vi "lv-ros-bridge_WRITE.vi"(10 "rosbridge port":u16=9090, 11 "rosbridge server IP":string="192.168.164.128") -> (0 "error out":errorcluster)   [LabVIEW 2015]
uses:
  Control  rossss.ctl
  <vilib>/Utility/inputDevices.llb/joystickAcquire.vi
  <vilib>/Utility/inputDevices.llb/closeJoystick.vi
  <vilib>/Intelligent Energy/WebSockets API/WebSockets/WebSockets.lvlib
panel:
  in  "ms to wait":u32=10
  in  "msg.layout.dim":T1(array[cluster])
  out "output cluster":T2={"op"="publish", "topic"="", "msg"={"layout"={"dim"=[], "data_offset"=0.0}, "data"=[]}}
  out "Opcode 2":u8
  out "Data 2":string
  out "concatenated string":string
  in  "type":string="std_msgs/Int32MultiArray"
  out "direction info":T3
  out "button info":T4
  out "axis info":T5
  in  "device index":i32
  in  "Topic to write":string="rio"
  in  "format wiadomości":T2={"op"="publish", "topic"="", "msg"={"layout"={"dim"=[], "data_offset"=0.0}, "data"=[]}}
  out "raw JSON frame":string
  in  "stop":bool
  # "ZAWSZE UŻYWAJ STOPU!!!"
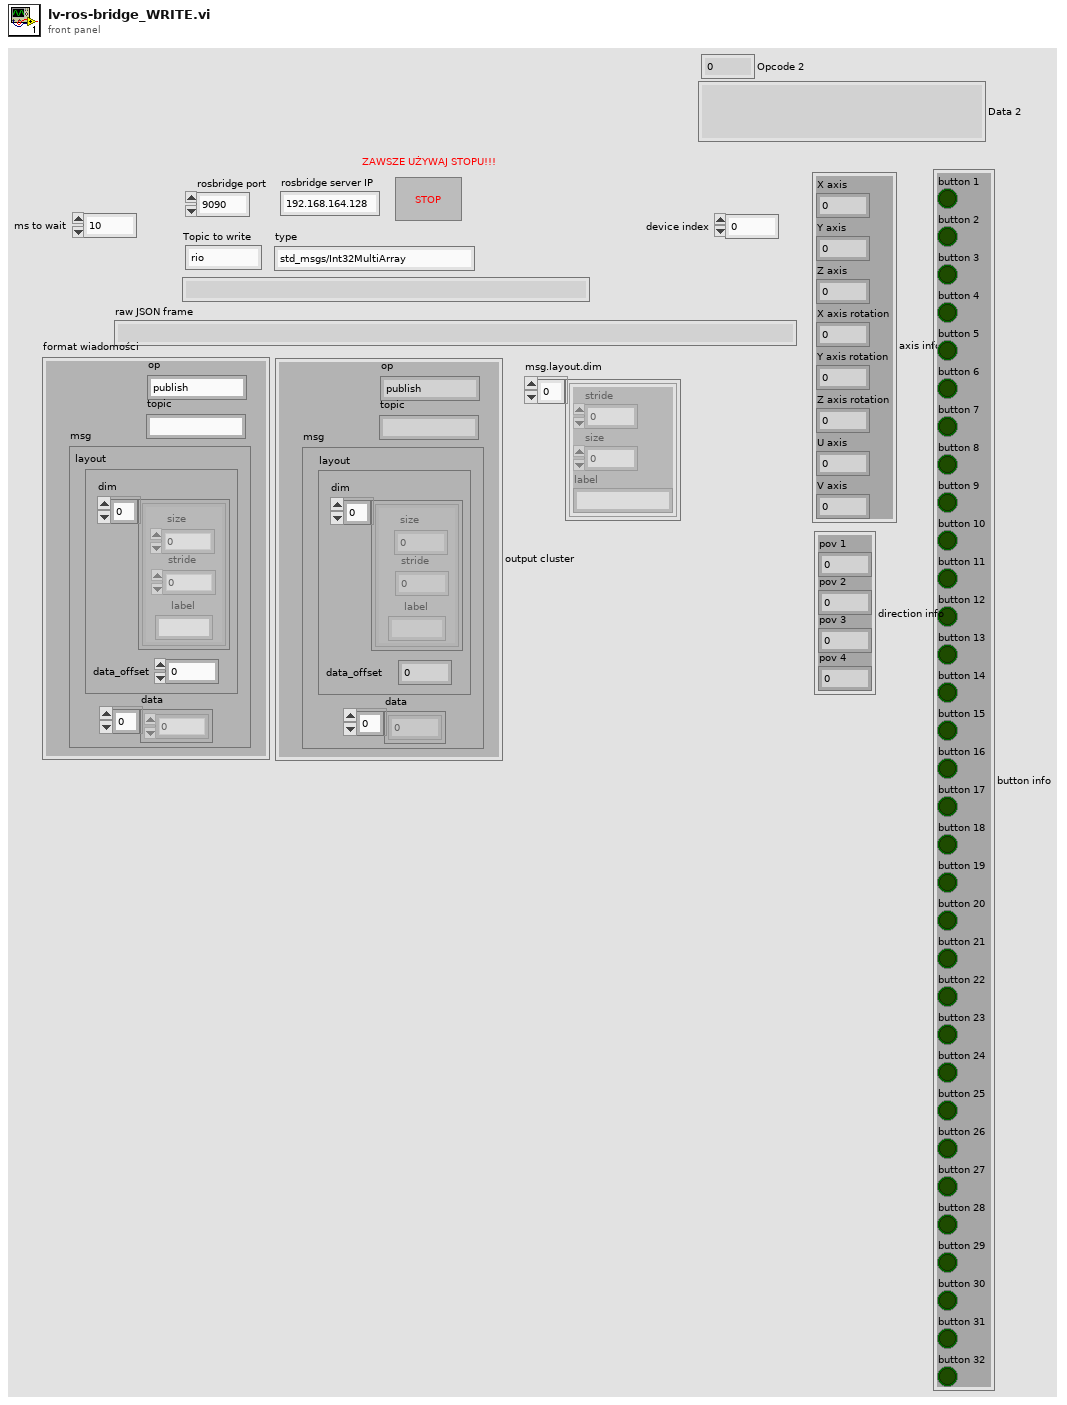
[diagram p1: front panel]
types:
  T1 = cluster{"stride":i16, "size":i16, "label":string}[]
  T2 = typedef "Control  rossss.ctl" = cluster{"op":string, "topic":string, "msg":cluster{"layout":cluster{"dim":cluster{"stride":i16, "size":i16, "label":string}[], "data_offset":dbl}, "data":i32[]}}
  T3 = cluster{"pov 1":i32, "pov 2":i32, "pov 3":i32, "pov 4":i32}
  T4 = cluster{"button 1":bool, "button 2":bool, "button 3":bool, "button 4":bool, "button 5":bool, "button 6":bool, "button 7":bool, "button 8":bool, "button 9":bool, "button 10":bool, "button 11":bool, "button 12":bool, "button 13":bool, "button 14":bool, "button 15":bool, "button 16":bool, "button 17":bool, "button 18":bool, "button 19":bool, "button 20":bool, "button 21":bool, "button 22":bool, "button 23":bool, "button 24":bool, "button 25":bool, "button 26":bool, "button 27":bool, "button 28":bool, "button 29":bool, "button 30":bool, "button 31":bool, "button 32":bool}
  T5 = cluster{"X axis":i32, "Y axis":i32, "Z axis":i32, "X axis rotation":i32, "Y axis rotation":i32, "Z axis rotation":i32, "U axis":i32, "V axis":i32}
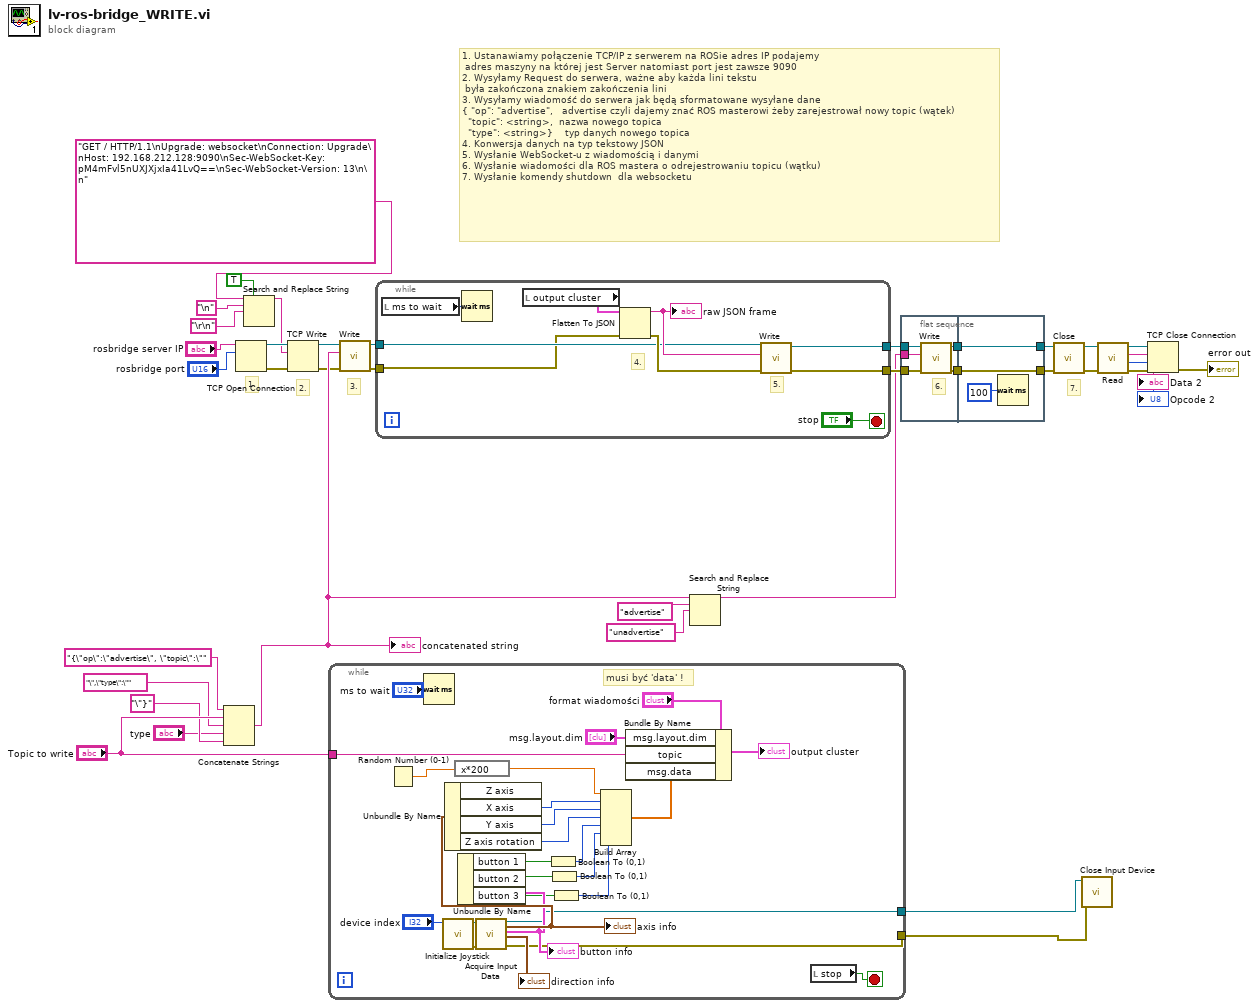
[diagram p0: block diagram]
diagram:
  # "1. Ustanawiamy połączenie TCP/IP z serwerem na ROSie adres IP podajemy\n adres maszyny na której jest Server natomiast port jest zawsze 9090\n2. Wysyłamy Request do serwera, ważne aby każda lini tekstu\n była zakończona znakiem zakończenia lini\n3. Wysyłamy wiadomość do serwera jak będą sformatowane wysyłane dane \n{ \"op\": \"advertise\",   advertise czyli dajemy znać ROS masterowi żeby zarejestrował nowy topic (wątek)\n  \"topic\": <string>,  nazwa nowego topica \n  \"type\": <string>}    typ danych nowego topica\n4. Konwersja danych na typ tekstowy JSON\n5. Wysłanie WebSocket-u z wiadomością i danymi\n6. Wysłanie wiadomości dla ROS mastera o odrejestrowaniu topicu (wątku)\n7. Wysłanie komendy shutdown  dla websocketu"
  # "7."
  # "3."
  # "2."
  # "1."
  n1 = Concatenate Strings("{\"op\":\"advertise\", \"topic\":\"", "Topic to write", "\",\"type\":\"", "type", "\"}") -> (w32:string)
  "concatenated string" <- w32
  n2 = TCP Open Connection(address="rosbridge server IP", remote port or service name="rosbridge port") -> (connection ID=w14:refnum<k5>, error out=w13:errorcluster)  [unwired: 3 in]
  n3 = Search and Replace String(replace all?=TRUE ("replace all? (F)"), input string="GET / HTTP/1.1\nUpgrade: websocket\nConnection: Upgrade\nHost: 192.168.212.128:9090\nSec-WebSocket-Key: pM4mFvl5nUXJXjxIa41LvQ==\nSec-WebSocket-Version: 13\n\n", search string="\n", replace string="\r\n") -> (result string=w12:string)  [unwired: 4 in, 3 out]
  n4 = TCP Write(connection ID=w14, data in=w12, error in (no error)=w13) -> (connection ID out=w2:refnum<k5>, error out=w1:errorcluster)  [unwired: 1 in, 1 out]
  n5 = while {
    tunnel: "Topic to write" -> [w61]
    tunnel: [w44] -> w31
    tunnel: [w43] -> w30
    stop <- w62 stop-if-true
    # "musi być 'data' !"
    n6 = Random Number (0-1)() -> (number: 0 to 1=w39:dbl)
    n7 = Wait (ms)(milliseconds to wait="ms to wait") -> ()  [unwired: 1 out]
    n8 = call <vilib>:"Initialize Joystick.vi"("device index"="device index") -> ("error out"=w56:errorcluster, "device ID"=w57:refnum<k1>)  [unwired: 9 in]
    n9 = expression code="x*200"(w39) -> (w38:dbl)
    n10 = call-poly <vilib>:"Acquire Input Data.vi"("device ID"=w57, "error in (no error)"=w56) -> ("device ID"=w44:refnum<k1>, "axis info"=w55:T5, "button info"=w51:T4, "direction info"=→"direction info":T3, "error out"=w43:errorcluster)  [unwired: 13 in]
    "axis info" <- w55
    "button info" <- w51
    n11 = Unbundle By Name(w55) -> ("X axis"=w54:i32, "Y axis"=w53:i32, "Z axis rotation"=w52:i32)  [unwired: 1 out]
    n12 = Unbundle By Name(w51) -> ("button 1"=w48:bool, "button 2"=w49:bool, "button 3"=w50:bool)
    n13 = Boolean To (0,1)(Boolean=w48) -> (0, 1=w47:i16)
    n14 = Boolean To (0,1)(Boolean=w49) -> (0, 1=w46:i16)
    n15 = Boolean To (0,1)(Boolean=w50) -> (0, 1=w45:i16)
    n16 = Build Array(w38, w54, w53, w52, w47, w46, w45) -> (w41:dbl[])
    n17 = Bundle By Name(cluster="format wiadomości", "msg.layout.dim"="msg.layout.dim", "topic"=w61, "msg.data"=w41) -> (→"output cluster":T2)
    n18 = local read "stop"() -> (w62:bool)
  }
  n19 = call <vilib>:"Write.vi"("error in (no error)"=w1, "Data"=w32, "WebSocket Connection in"=w2) -> ("error out"=w26:errorcluster, "WebSocket Connection out"=w25:refnum<k5>)  [unwired: 7 in]
  n20 = while {
    tunnel: [w72] -> w23
    tunnel: [w71] -> w21
    tunnel: w25 -> [w66]
    tunnel: w26 -> [w65]
    stop <- "stop" stop-if-true
    # "5."
    # "4."
    n21 = local read "ms to wait"() -> (w64:u32)
    n22 = Wait (ms)(milliseconds to wait=w64) -> ()  [unwired: 1 out]
    n23 = local read "output cluster"() -> (w68:T2)
    n24 = Flatten To JSON(anything=w68, error in (no error)=w65) -> (JSON string=w69:string, 11:w67:errorcluster)  [unwired: 1 in]
    "raw JSON frame" <- w69
    n25 = call <vilib>:"Write.vi"("error in (no error)"=w67, "Data"=w69, "WebSocket Connection in"=w66) -> ("error out"=w71:errorcluster, "WebSocket Connection out"=w72:refnum<k5>)  [unwired: 7 in]
  }
  n26 = Search and Replace String(input string=w32, search string="advertise", replace string="unadvertise" ("search string")) -> (result string=w11:string)  [unwired: 5 in, 3 out]
  n27 = flat-sequence {
    tunnel: w23 -> [w77]
    tunnel: w21 -> [w76]
    tunnel: w11 -> [w75]
    tunnel: [w74] -> w29
    tunnel: [w73] -> w28
    tunnel: [w79] -> w22
    tunnel: [w80] -> w24
    tunnel: w29 -> [w80]
    tunnel: w28 -> [w79]
    frame #0 {
      # "6."
      n28 = call <vilib>:"Write.vi"("error in (no error)"=w76, "Data"=w75, "WebSocket Connection in"=w77) -> ("error out"=w73:errorcluster, "WebSocket Connection out"=w74:refnum<k5>)  [unwired: 7 in]
    }
    frame #1 {
      n29 = Wait (ms)(milliseconds to wait=u32 100) -> ()  [unwired: 1 out]
    }
  }
  n30 = call <vilib>:"Close.vi"("error in (no error)"=w22, "WebSocket Connection in"=w24) -> ("error out"=w7:errorcluster, "WebSocket Connection in"=w8:refnum<k5>)  [unwired: 8 in]
  n31 = call-poly <vilib>:"Close Input Device.vi"("error in (no error)"=w30, "device ID"=w31) -> ()  [unwired: 8 in, 1 out]
  n32 = call <vilib>:"Read.vi"("error in (no error)"=w7, "WebSocket Connection in"=w8) -> ("error out"=w6:errorcluster, "Opcode"=→"Opcode 2":u8, "Data"=→"Data 2":string, "WebSocket Connection out"=w5:refnum<k5>)  [unwired: 6 in]
  n33 = TCP Close Connection(connection ID=w5, error in (no error)=w6) -> (error out=→"error out":errorcluster)  [unwired: 1 in, 1 out]
